vi "State Vector - Read.vi"(7 "QuWire in":refnum<class "QuWire.lvclass">) -> (8 "State Vector":cdb[](array[numeric]))   [LabVIEW 2020]
uses:
  QuSim/QuWire/QuWire.lvclass
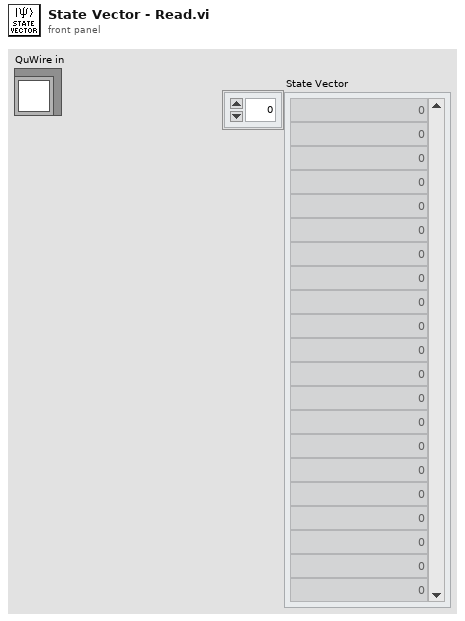
[diagram p1: front panel]
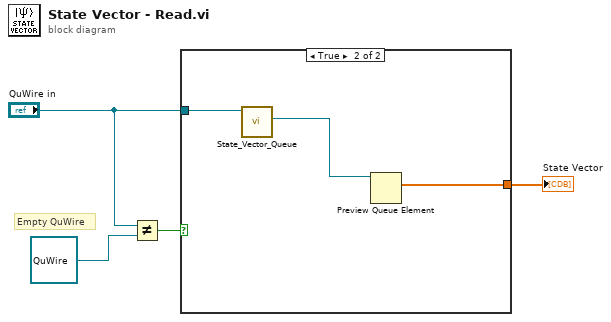
[diagram p0: block diagram]
diagram:
  # "Empty QuWire"
  n1 = Not Equal?(x="QuWire in", y=refnum<class "QuWire.lvclass"> refnum ("QuWire in")) -> (x != y?=w2:bool)
  n2 = case shown="True" w2 {
    tunnel: "QuWire in" -> [_ w5]
    tunnel: [_ w6] -> w1
    frame False {
    }
    frame True {
      n3 = call "State_Vector_Queue.vi"("QuWire in"=w5) -> ("State Vector Queue"=w7:refnum<queue>)  [unwired: 8 in, 2 out]
      n4 = Preview Queue Element(queue=w7) -> (element=w6:cdb[])  [unwired: 2 in, 3 out]
    }
  }
  "State Vector" <- w1
